vi "ArmAbsolutePoseToXYPoint_Array.vi"(1 "ArmAbsolutePose":T2[](array[typedef])) -> (0 "2DPoint":T1[](array[typedef]))   [LabVIEW 2018]
uses:
  TypeDefs/ArmAbsolutePosition.ctl
  ArgosLib/Path Planning/TypeDefs/Point2D.ctl
  ArgosLib/ArgosLib.lvlib
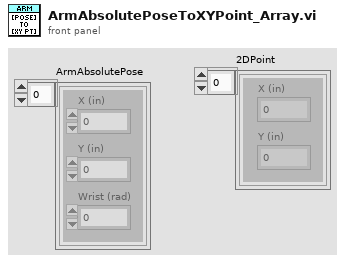
[diagram p1: front panel]
types:
  T1 = typedef "ArgosLib.lvlib/Point2D.ctl" = cluster{"X (in)":dbl, "Y (in)":dbl}
  T2 = typedef "ArmAbsolutePosition.ctl" = cluster{"X (in)":dbl, "Y (in)":dbl, "Wrist (rad)":dbl}
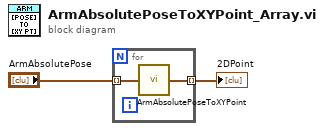
[diagram p0: block diagram]
diagram:
  n1 = for {
    tunnel: "ArmAbsolutePose" -> [w4] mode=indexing
    tunnel: [w3] -> w1 mode=indexing
    n2 = call "ArmAbsolutePoseToXYPoint.vi"("ArmAbsolutePose"=w4) -> ("2DPoint"=w3:T1)
  }
  "2DPoint" <- w1
